vi "Configure Offset And Limits List (Adjacent Channel Power).vi"(0 "VISA resource name":refnum<visa-resource-name>, 1 "Reference Bandwidth":dbl[](array[numeric])=[10000000.0, 10000000.0] format="%#.6g", 2 "Positive Offset Limit":dbl[](array[numeric])=[0.0, 0.0] format="%#.6g", 3 "Negative Offset Limit":dbl[](array[numeric])=[0.0, 0.0] format="%#.6g", 5 "Enable Frequency Offsets":bool[](array[boolean])=[TRUE, TRUE], 7 "Frequency Offsets":dbl[](array[numeric])=[10000000.0, 10000000.0] format="%#.6g", 11 "error in (no error)":errorcluster) -> (4 "VISA resource name out":refnum<visa-resource-name>, 15 "error out":errorcluster)   [LabVIEW 2014, in "Agilent ESA PSA Series.lvlib"]
doc: "Sets up offsets and limits of the adjacent channel power measurement operation."
uses:
  Agilent ESA PSA Series.lvlib
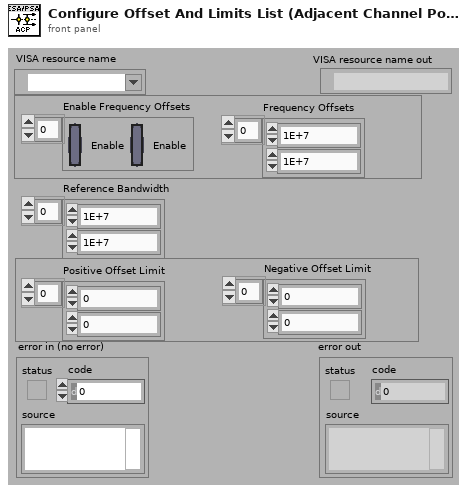
[diagram p1: front panel]
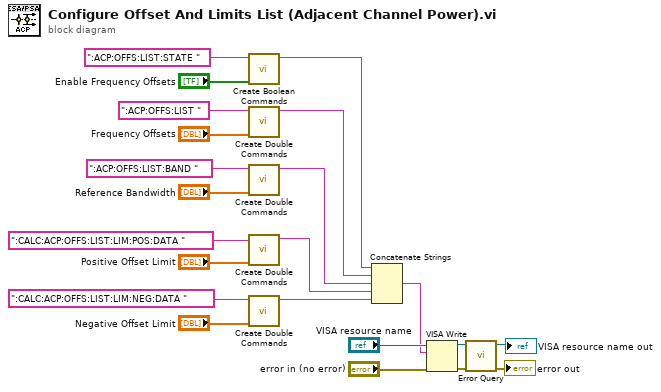
[diagram p0: block diagram]
diagram:
  n1 = call "Create Boolean Commands.vi"("States"="Enable Frequency Offsets", "Command"=":ACP:OFFS:LIST:STATE ") -> ("Result String"=w5:string)  [unwired: 9 in]
  n2 = call "Create Double Commands.vi"("Double Values"="Frequency Offsets", "Commands"=":ACP:OFFS:LIST ") -> ("Result"=w4:string)  [unwired: 9 in]
  n3 = call "Create Double Commands.vi"("Double Values"="Reference Bandwidth", "Commands"=":ACP:OFFS:LIST:BAND ") -> ("Result"=w3:string)  [unwired: 9 in]
  n4 = call "Create Double Commands.vi"("Double Values"="Positive Offset Limit", "Commands"=":CALC:ACP:OFFS:LIST:LIM:POS:DATA ") -> ("Result"=w2:string)  [unwired: 9 in]
  n5 = call "Create Double Commands.vi"("Double Values"="Negative Offset Limit", "Commands"=":CALC:ACP:OFFS:LIST:LIM:NEG:DATA ") -> ("Result"=w1:string)  [unwired: 9 in]
  n6 = Concatenate Strings(w5, w4, w3, w2, w1) -> (w16:string)
  n7 = VISA Write(VISA resource name="VISA resource name", write buffer=w16, error in (no error)="error in (no error)") -> (VISA resource name out=w21:refnum<visa-resource-name>, error out=w22:errorcluster)  [unwired: 1 out]
  n8 = call "Error Query.vi"("error in (no error)"=w22, "VISA resource name"=w21) -> ("error out"=→"error out":errorcluster, "VISA resource name out"=→"VISA resource name out":refnum<visa-resource-name>)  [unwired: 6 in, 2 out]
